vi "Start Timer.vi"(11 "Wait\nTime":dbl) -> (3 "Elapsed Time":dbl)   [LabVIEW 2019]
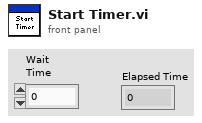
[diagram p1: front panel]
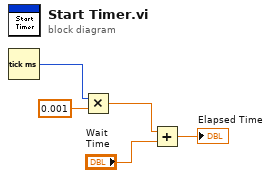
[diagram p0: block diagram]
diagram:
  n1 = Tick Count (ms)() -> (millisecond timer value=w4:u32)
  n2 = Multiply(x=w4, y=0.001) -> (x*y=w3:dbl)
  n3 = Add(x=w3, y="Wait\nTime") -> (x+y=→"Elapsed Time":dbl)
